vi "Generate Error.vi"(8 "Error In":errorcluster, 9 "Custom":T1, 11 "Enum":T2(ring)) -> (0 "Error Out":errorcluster)   [LabVIEW 2015]
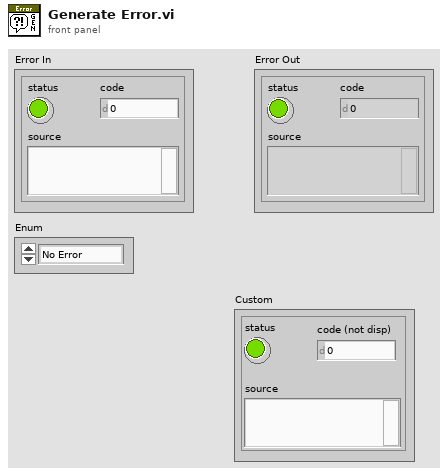
[diagram p1: front panel]
types:
  T1 = cluster{"status":bool, "code (not disp)":i32, "source":string}
  T2 = enum16{"No Error", "Custom", "Standard", "GPS Signal", "YH Left", "YL Right", "XL Back", "XH Front"}
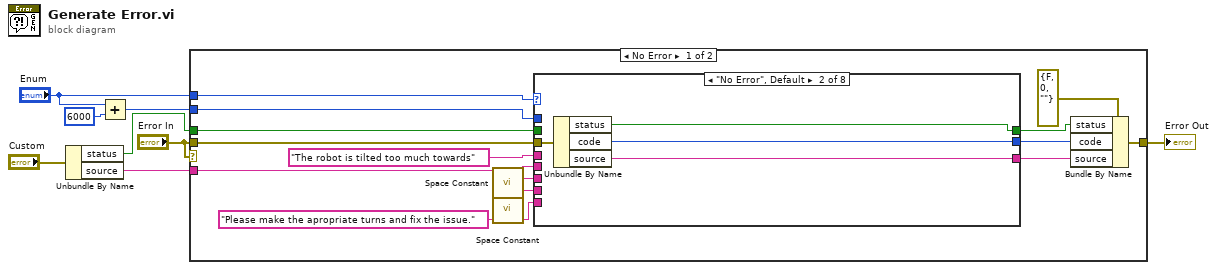
[diagram p0: block diagram]
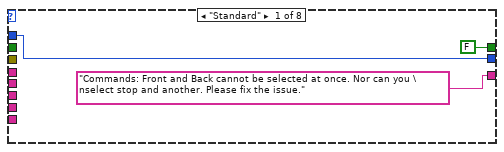
[diagram p2: hidden frame]
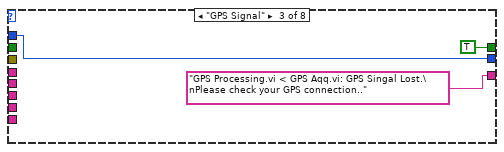
[diagram p3: hidden frame]
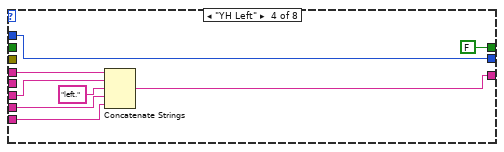
[diagram p4: hidden frame]
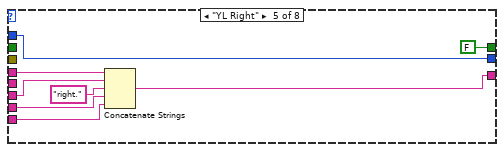
[diagram p5: hidden frame]
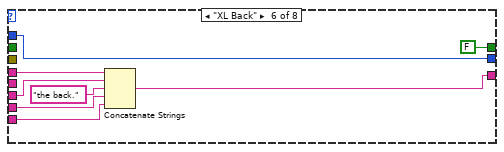
[diagram p6: hidden frame]
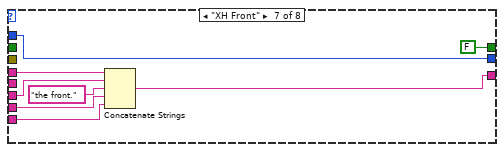
[diagram p7: hidden frame]
diagram:
  n1 = Unbundle By Name("Custom") -> ("status"=w1:bool, "source"=w2:string)
  n2 = Add(x="Enum", y=6000) -> (x+y=w8:i32)
  n3 = case shown="No Error" "Error In" {
    tunnel: "Enum" -> [w17 _]
    tunnel: w2 -> [w22 _]
    tunnel: w8 -> [w21 _]
    tunnel: [w16 w68] -> w5
    tunnel: "Error In" -> [w14 w68]
    tunnel: w1 -> [w13 _]
    frame No Error {
      n4 = call <vilib>:"Space Constant.vi"() -> ("String"=w11:string)
      n5 = call <vilib>:"Space Constant.vi"() -> ("String"=w9:string)
      n6 = case shown="\"No Error\", Default" w17 {
        tunnel: w22 -> [_ _ _ _ _ _ _ w67]
        tunnel: w21 -> [w24 _ w32 w39 w47 w55 w63 w66]
        tunnel: [w24 w27 w32 w39 w47 w55 w63 w66] -> w19
        tunnel: ["Commands: Front and Back cannot be selected at once. Nor can you \nselect stop and another. Please fix the issue." ("source") w26 "GPS Processing.vi < GPS Aqq.vi: GPS Singal Lost.\nPlease check your GPS connection.." ("Description") w34 w42 w50 w58 w67] -> w18
        tunnel: [FALSE ("status") w28 TRUE ("status") FALSE ("status") FALSE ("status") FALSE ("status") FALSE ("status") w65] -> w15
        tunnel: w14 -> [_ w29 _ _ _ _ _ _]
        tunnel: w13 -> [_ _ _ _ _ _ _ w65]
        tunnel: "The robot is tilted too much towards" ("source") -> [_ _ _ w38 w46 w54 w62 _]
        tunnel: w11 -> [_ _ _ w37 w45 w53 w61 _]
        tunnel: "Please make the apropriate turns and fix the issue." ("source") -> [_ _ _ w35 w43 w51 w59 _]
        tunnel: w9 -> [_ _ _ w36 w44 w52 w60 _]
        frame "Standard" {
        }
        frame "No Error", Default {
          n7 = Unbundle By Name(w29) -> ("status"=w28:bool, "code"=w27:i32, "source"=w26:string)
        }
        frame "GPS Signal" {
        }
        frame "YH Left" {
          n8 = Concatenate Strings(w38, w37, "left." ("string"), w36, w35) -> (w34:string)
        }
        frame "YL Right" {
          n9 = Concatenate Strings(w46, w45, "right." ("string"), w44, w43) -> (w42:string)
        }
        frame "XL Back" {
          n10 = Concatenate Strings(w54, w53, "the back." ("string"), w52, w51) -> (w50:string)
        }
        frame "XH Front" {
          n11 = Concatenate Strings(w62, w61, "the front." ("string"), w60, w59) -> (w58:string)
        }
        frame "Custom" {
        }
      }
      n12 = Bundle By Name(cluster=errorcluster {"status"=FALSE, "code"=0, "source"=""} ("error constant"), "status"=w15, "code"=w19, "source"=w18) -> (w16:errorcluster)
    }
    frame Error {
    }
  }
  "Error Out" <- w5
